vi "1. Histogram, Color Space and Threshold.vi"() -> ()   [LabVIEW 2019]
doc: "c 2020 ReMiSYS All rights reserved."
panel:
  in  "offset":i32(slide)=29 scale=0.0..50.0
  in  "Color Mode":enum16{"RGB", "HSL", "HSV", "HSI"}(ring)
  in  "Manual Threshold?":bool
  in  "Blue or Luminance":cluster{i32, i32}(slide)={20, 217} scale=0.0..255.0
  in  "Green or Saturation":cluster{i32, i32}(slide)={20, 233} scale=0.0..255.0
  in  "Red or Hue":cluster{i32, i32}(slide)={42, 99} scale=0.0..255.0
  out "Histogram Graph":u32[][](graph)
  out "Bin Image":T1(plugin-control)
  out "Ori Image":T1(plugin-control)
  in  "Stop (F)":bool
  # "Minimum"
  # "Maximum"
  # "Minimum"
  # "Maximum"
  # "Minimum"
  # "Maximum"
  # "c 2022 ReMiSYS All rights reserved."
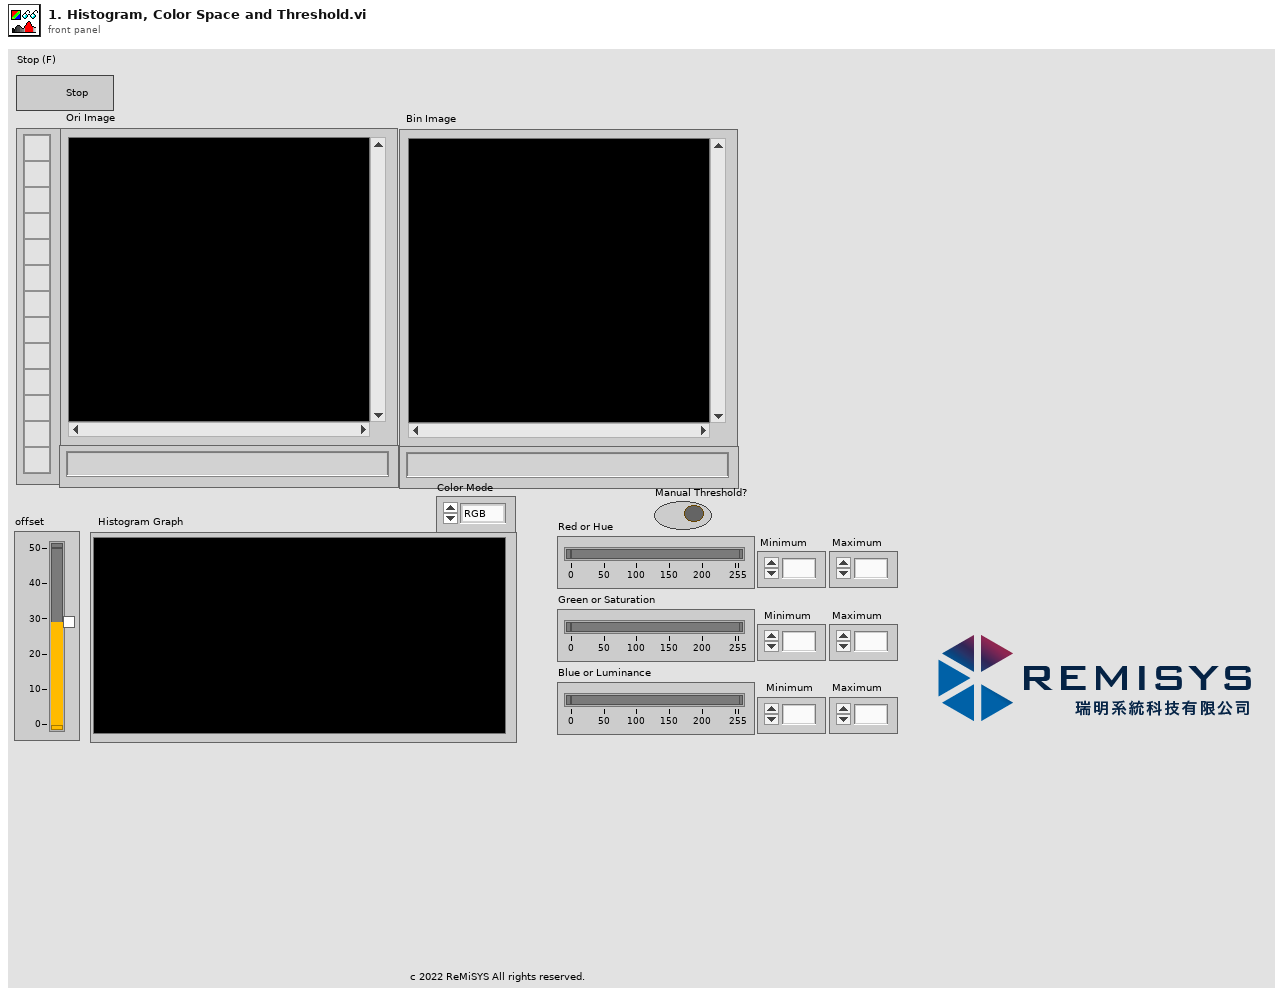
[diagram p1: front panel]
types:
  T1 = typedef "IMAQ Image.ctl" = refnum<image>
  T2 = cluster{"Cluster":cluster{"Numeric Control":i32, "Numeric Control":i32}, "Cluster":cluster{"Numeric Control":i32, "Numeric Control":i32}, "Cluster":cluster{"Numeric Control":i32, "Numeric Control":i32}}
  T3 = cluster{"Numeric Control":i32, "Numeric Control":i32}
  T4 = cluster{"Global Rectangle":i32[], "Contours":cluster{"Contour Type":u32, "ROI Type":u32, "Points":i32[]}[]}
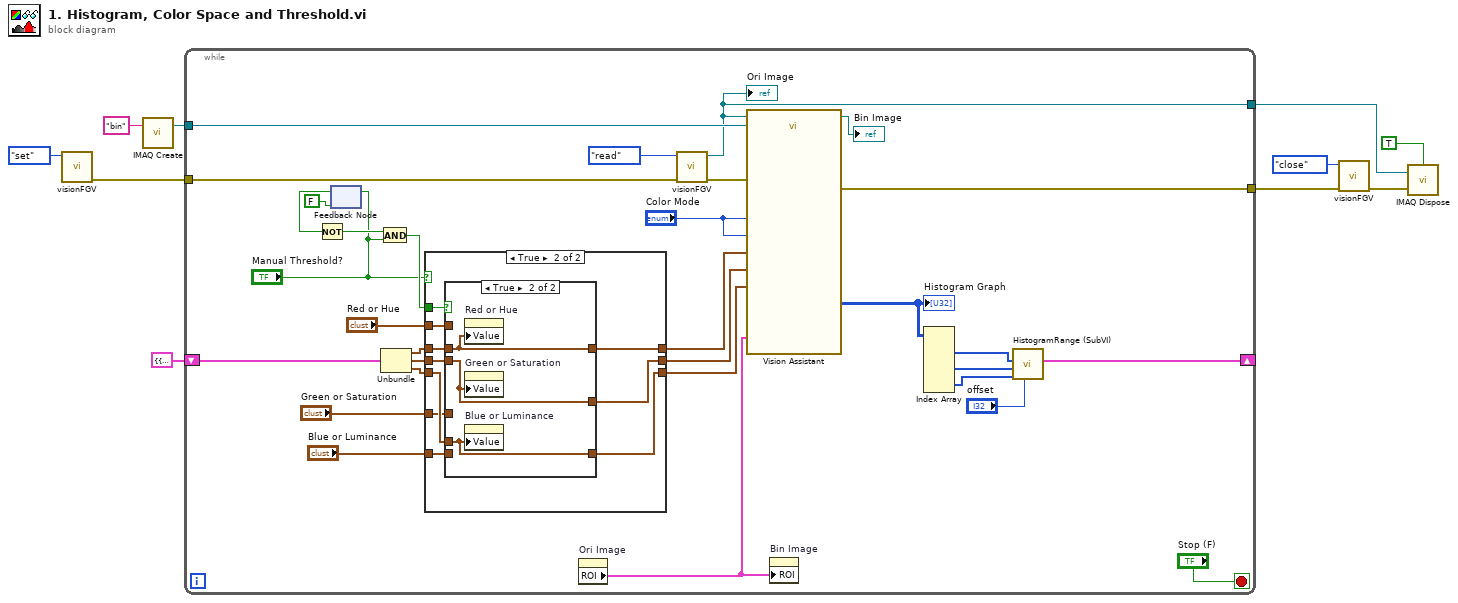
[diagram p0: block diagram]
diagram:
  n1 = call "visionFGV.vi"("Function"=enum16{"set", "read", "close"}."set") -> ("error out"=w5:errorcluster)  [unwired: 9 in, 1 out]
  n2 = call "IMAQ Create"("Image Name"="bin") -> ("New Image"=w8:T1)  [unwired: 4 in, 1 out]
  n3 = while {
    tunnel: [w40] -> w10
    tunnel: w8 -> [w41]
    shift-right: [w22] -> _
    shift-left: T2 {"Cluster"={"Numeric Control"=0, "Numeric Control"=0}, "Cluster"={"Numeric Control"=0, "Numeric Control"=0}, "Cluster"={"Numeric Control"=0, "Numeric Control"=0}} ("Output Range") -> [w23]
    tunnel: w5 -> [w14]
    tunnel: [w12] -> w1
    stop <- "Stop (F)" stop-if-true
    n4 = feedback #1(FALSE ("Manual Threshold?")) -> (w30:bool)
    n5 = Not(x=w30) -> (.not. x?=w17:bool)
    n6 = feedback-in #1("Manual Threshold?") -> ()
    n7 = And(x=w17, y="Manual Threshold?") -> (x .and. y?=w31:bool)
    n8 = Unbundle(w23) -> ("Cluster"=w26:T3, "Cluster"=w25:T3, "Cluster"=w24:T3)
    n9 = case shown="True" "Manual Threshold?" {
      tunnel: [w44 w54] -> w37
      tunnel: [w43 w53] -> w36
      tunnel: [w42 w52] -> w35
      tunnel: w26 -> [w44 w50]
      tunnel: w25 -> [w43 w48]
      tunnel: w24 -> [w42 w49]
      tunnel: w31 -> [_ w51]
      tunnel: "Blue or Luminance" -> [_ w47]
      tunnel: "Green or Saturation" -> [_ w46]
      tunnel: "Red or Hue" -> [_ w45]
      frame False {
      }
      frame True {
        n10 = case shown="True" w51 {
          tunnel: [w55 w60] -> w54
          tunnel: [w56 w58] -> w53
          tunnel: [w57 w59] -> w52
          tunnel: w50 -> [_ w60]
          tunnel: w49 -> [_ w59]
          tunnel: w48 -> [_ w58]
          tunnel: w47 -> [w57 _]
          tunnel: w46 -> [w56 _]
          tunnel: w45 -> [w55 _]
          frame False {
          }
          frame True {
            n11 = property on="Red or Hue" class="Slide (strict)"("Value"=w60) -> ()  [unwired: 2 in, 2 out]
            n12 = property on="Green or Saturation" class="Slide (strict)"("Value"=w58) -> ()  [unwired: 2 in, 2 out]
            n13 = property on="Blue or Luminance" class="Slide (strict)"("Value"=w59) -> ()  [unwired: 2 in, 2 out]
          }
        }
      }
    }
    n14 = property on="Ori Image" class="ImageControl"() -> ("ROI"=w38:T4)  [unwired: 2 in, 2 out]
    n15 = call "visionFGV.vi"("Error In"=w14, "Function"=enum16{"set", "read", "close"}."read") -> ("error out"=w11:errorcluster, "Image Out fgv"=w40:T1)  [unwired: 8 in]
    "Ori Image" <- w40
    n16 = call "Vision Assistant"("Image In"=w40, "Image Dst"=w41, "Color Mode (Histogram 1)"="Color Mode", "Color Mode (Color Threshold 1)"="Color Mode", "Red or Hue Range (Color Threshold 1)"=w37, "Green or Sat Range (Color Threshold 1)"=w36, "Blue or Luma or Val or Inten Range (Color Threshold 1)"=w35, "error in"=w11, "ROI Descriptor (Histogram 1)"=w38) -> ("Image Out"=→"Bin Image":T1, "Histogram (Histogram 1)"=w33:u32[][], "error out"=w12:errorcluster)  [unwired: 15 in, 1 out]
    "Histogram Graph" <- w33
    n17 = property on="Bin Image" class="ImageControl"("ROI"=w38) -> ()  [unwired: 2 in, 2 out]
    n18 = Index Array(array=w33) -> (element #1=w32:u32[], element #2=w28:u32[], element #3=w27:u32[])  [unwired: 6 in]
    n19 = call "HistogramRange (SubVI).vi"("offset"="offset", "Histogram Graph3"=w27, "Histogram Graph2"=w28, "Histogram Graph1"=w32) -> ("Output Range"=w22:T2)  [unwired: 7 in]
  }
  n20 = call "visionFGV.vi"("Error In"=w1, "Function"=enum16{"set", "read", "close"}."close") -> ("error out"=w2:errorcluster)  [unwired: 8 in, 1 out]
  n21 = call "IMAQ Dispose"("All Images? (No)"=TRUE, "Image"=w10, "error in (no error)"=w2) -> ()  [unwired: 3 in, 1 out]
